vi "Lang Set Desc other.vi"(8 "error in (no error)":errorcluster, 10 "Other":T1, 11 "LF2R IDE in":refnum<class "Main Panel.lvclass">) -> (0 "error out":errorcluster, 3 "LF2R IDE out":refnum<class "Main Panel.lvclass">)   [LabVIEW 2018, in "Framework.lvlib" / "Framework.lvclass"]
uses:
  Framework/Framework/Framework.lvclass
  Main Panel.lvclass
  D:/project/hobby/LabVIEW/LF2R/LabVIEW/Source/Actor/Framework/Framework/Framework.lvclass
  C:/Program Files (x86)/National Instruments/LabVIEW 2018/vi.lib/MGI/Panel Manager/Panel Actor/Panel Actor/Panel Actor.lvclass
  C:/Program Files (x86)/National Instruments/LabVIEW 2018/vi.lib/MGI/Monitored Actor/Monitored Actor/Monitored Actor/Monitored Actor.lvclass
  C:/Program Files (x86)/National Instruments/LabVIEW 2018/vi.lib/ActorFramework/Actor/Actor.lvclass
  Const Lang Property.ctl
  Const UI Desc Other.ctl
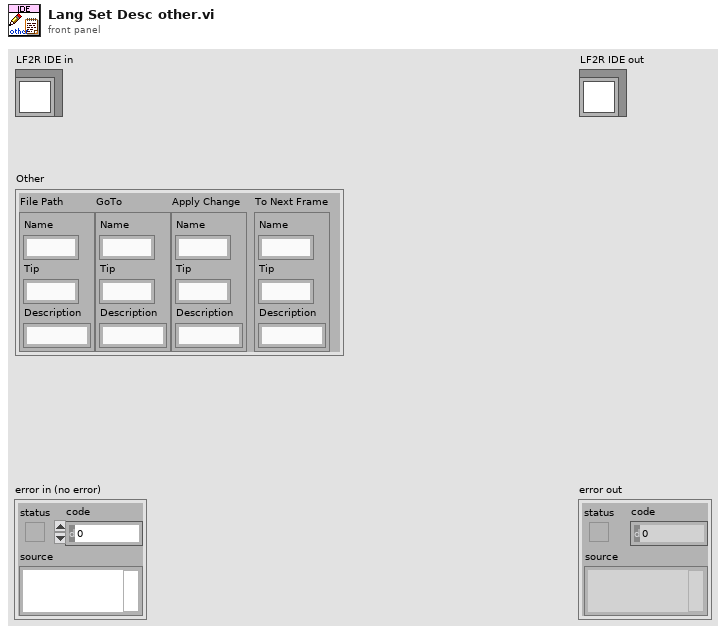
[diagram p1: front panel]
types:
  T1 = typedef "Framework.lvlib/Framework.lvclass/Const UI Desc Other.ctl" = cluster{"File Path":T2, "GoTo":T2, "Apply Change":T2, "To Next Frame":T2}
  T2 = typedef "Framework.lvlib/Framework.lvclass/Const Lang Property.ctl" = cluster{"Name":string, "Tip":string, "Description":string}
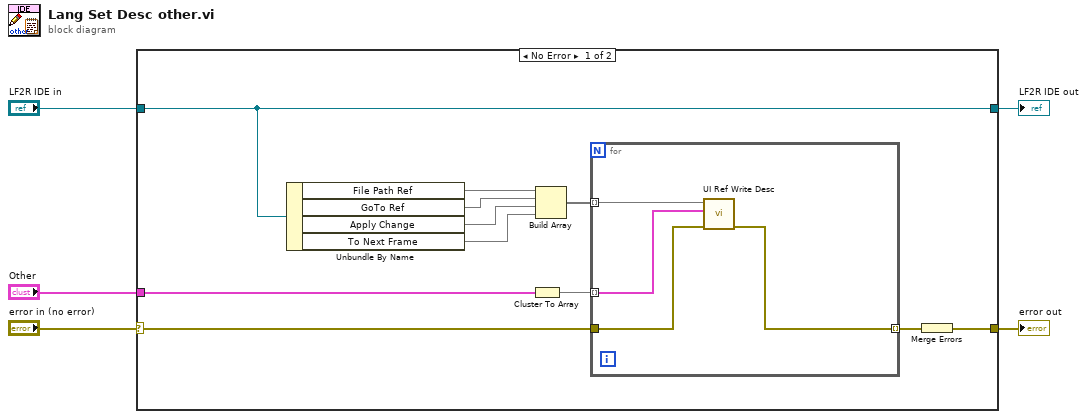
[diagram p0: block diagram]
diagram:
  n1 = case shown="No Error" "error in (no error)" {
    selector: "error in (no error)" -> [w14 w22]
    tunnel: [w13 w22] -> w4
    tunnel: [w16 w21] -> w2
    tunnel: "LF2R IDE in" -> [w16 w21]
    tunnel: "Other" -> [w15 _]
    frame No Error {
      n2 = Unbundle By Name(w16) -> ("File Path Ref"=w9, "GoTo Ref"=w8, "Apply Change"=w7, "To Next Frame"=w6)
      n3 = Cluster To Array(cluster=w15) -> (array=w11:T2[])
      n4 = Build Array(w9, w8, w7, w6) -> (w12:void[])
      n5 = for {
        tunnel: w12 -> [w17] mode=indexing
        tunnel: w11 -> [w20] mode=indexing
        tunnel: w14 -> [w19]
        tunnel: [w18] -> w10 mode=indexing
        n6 = call "UI Ref Write Desc.vi"("error in (no error)"=w19, "UI Property"=w20, "UI Ref"=w17) -> ("error out"=w18:errorcluster)  [unwired: 8 in]
      }
      n7 = Merge Errors(w10) -> (w13:errorcluster)
    }
    frame Error {
    }
  }
  "error out" <- w4
  "LF2R IDE out" <- w2
